vi "Read configuration.vi"(8 "error in":errorcluster, 11 "Convert Bool to Velocity editor node in":refnum<class "Convert Bool to Velocity editor node.lvclass">) -> (0 "error out":errorcluster, 2 "configuration":refnum<class "NISE_CEF_serializable configuration.lvclass">, 3 "Convert Bool to Velocity editor node out":refnum<class "Convert Bool to Velocity editor node.lvclass">)   [LabVIEW 2017, in "Convert Bool to Velocity editor node.lvclass"]
uses:
  Convert Bool to Velocity editor node.lvclass
  <vilib>/NI/Configuration Framework/serializable configuration/NISE_CEF_serializable configuration.lvclass
  Convert Bool to Velocity editor node.lvclass/Convert Bool to Velocity editor node.ctl
  module/configuration/Convert Bool to Velocity configuration.lvclass
  C:/Program Files (x86)/National Instruments/LabVIEW 2017/vi.lib/NI/Configuration Framework/serializable configuration/NISE_CEF_serializable configuration.lvclass
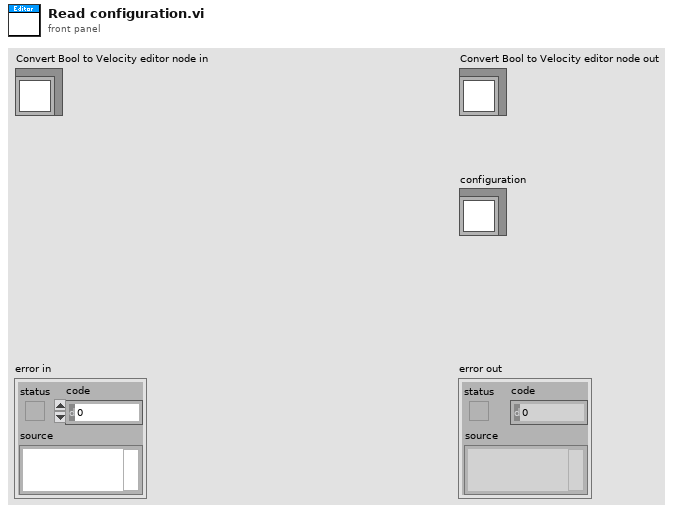
[diagram p1: front panel]
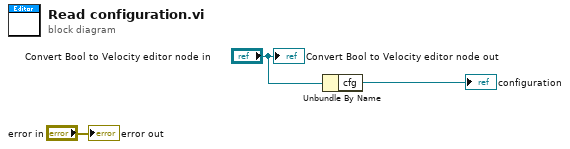
[diagram p0: block diagram]
diagram:
  n1 = Unbundle By Name("Convert Bool to Velocity editor node in") -> ("cfg"=→"configuration":refnum<class "Convert Bool to Velocity configuration.lvclass">)
  "error out" <- "error in"
  "Convert Bool to Velocity editor node out" <- "Convert Bool to Velocity editor node in"
